vi "Create Sample Clock.vi"(8 "error in (no error)":errorcluster, 11 "DAQmx in":refnum<class "DAQmx.lvclass">) -> (0 "error out":errorcluster, 3 "DAQmx out":refnum<class "DAQmx.lvclass">)   [LabVIEW 2019, in "DAQmx.lvclass"]
uses:
  DAQmx.lvclass
  <resource>/objmgr/daqmx.rc
  <vilib>/DAQmx/configure/timing.llb/DAQmx Timing (Sample Clock).vi
  typedefs/DAQ.Config.Sampling.Sampling--Cluster.ctl
panel:
  out "Sampling":T1={"Fs"=204789.0, "#s"=15753} {"Fs" format="%#_13g"}
  out "Fs (S/s) 3":dbl[](array[numeric]) format="%#_13g"
  out "Fs (S/s) 2":dbl[](array[numeric]) format="%#_13g"
  out "Output.Onboard Buffer":u32[](array[numeric])
  out "Output.Buffer":u32[](array[numeric])
  out "Input.Onboard Buffer":u32[](array[numeric])
  out "Input.Buffer":u32[](array[numeric])
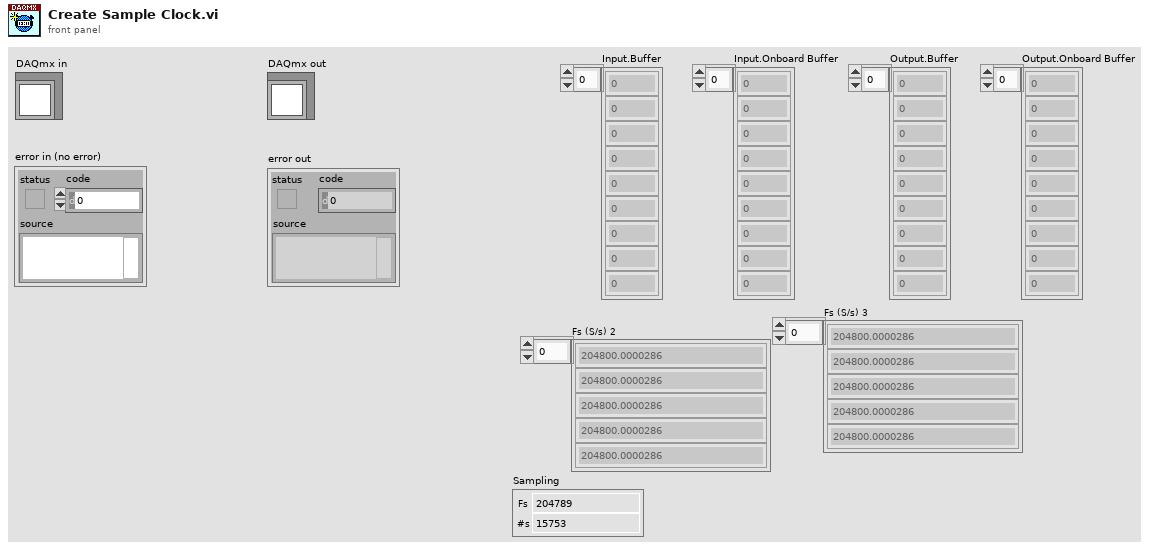
[diagram p1: front panel]
types:
  T1 = typedef "DAQmx.lvclass/DAQ.Config.Sampling.Sampling--Cluster.ctl" = cluster{"Fs":dbl, "#s":i32}
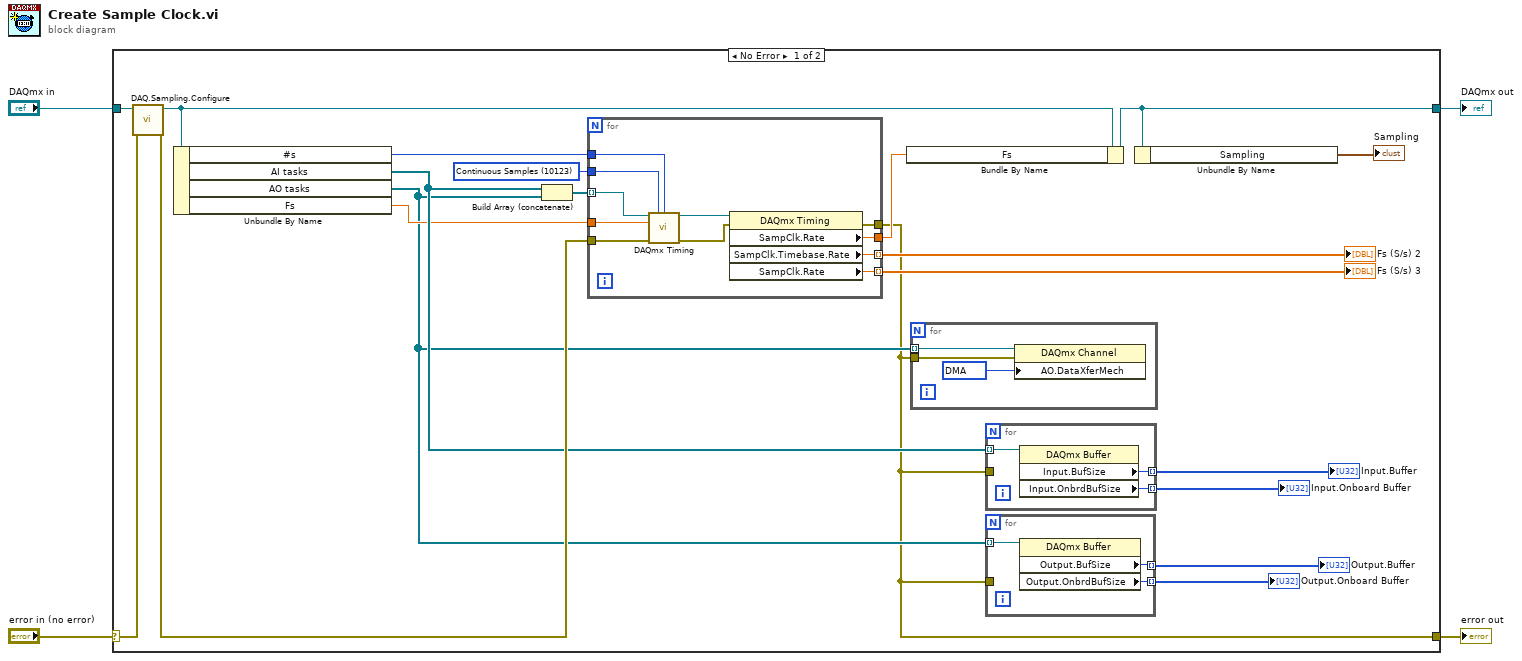
[diagram p0: block diagram]
diagram:
  n1 = case shown="No Error" "error in (no error)" {
    selector: "error in (no error)" -> [w14 w46]
    tunnel: [w5 w46] -> w4
    tunnel: [w9 w45] -> w2
    tunnel: "DAQmx in" -> [w24 w45]
    frame No Error {
      w8 = 10123 items=["Finite Samples"=10178, "Continuous Samples"=10123, "Hardware Timed Single Point"=12522] ("sample mode")
      n2 = call "DAQ.Sampling.Configure.vi"("error in (no error)"=w14, "DAQmx in"=w24) -> ("error out"=w22:errorcluster, "DAQmx out"=w23:refnum<class "DAQmx.lvclass">)  [unwired: 7 in, 1 out]
      n3 = Unbundle By Name(w23) -> ("#s"=w15:i32, "AI tasks"=w16:refnum<k21>[], "AO tasks"=w7:refnum<k21>[], "Fs"=w13:dbl)
      n4 = Build Array (concatenate)(w16, w7) -> (w21:refnum<k21>[])
      n5 = for {
        tunnel: w21 -> [w33] mode=indexing
        tunnel: w13 -> [w32]
        tunnel: w22 -> [w31]
        tunnel: [w35] -> w5
        tunnel: [w37] -> w12
        tunnel: w15 -> [w34]
        tunnel: [w30] -> w11 mode=indexing
        tunnel: [w29] -> w10 mode=indexing
        tunnel: w8 -> [w28]
        n6 = call-poly <vilib>:"DAQmx Timing.vi"("task/channels in"=w33, "sample mode"=w28, "samples per channel"=w34, "rate"=w32, "error in"=w31) -> ("task out"=w38:refnum<k21>, "error out"=w36:errorcluster)  [unwired: 9 in]
        n7 = property class="DAQmx Timing"(reference=w38, error in=w36) -> (error out=w35:errorcluster, "SampClk.Rate"=w37:dbl, "SampClk.Timebase.Rate"=w30:dbl, "SampClk.Rate"=w29:dbl)  [unwired: 1 out]
      }
      "Fs (S/s) 2" <- w11
      "Fs (S/s) 3" <- w10
      n8 = Bundle By Name(cluster=w23, "Fs"=w12) -> (w9:refnum<class "DAQmx.lvclass">)
      n9 = for {
        tunnel: w7 -> [w27] mode=indexing
        tunnel: w5 -> [w26]
        w25 = 10054 items=["DMA"=10054, "Interrupts"=10204, "Programmed I/O"=10264, "USB Bulk"=12590] ("AO.DataXferMech")
        n10 = property class="DAQmx Channel"(reference=w27, error in=w26, "AO.DataXferMech"=w25) -> ()  [unwired: 2 out]
      }
      n11 = for {
        tunnel: w16 -> [w44] mode=indexing
        tunnel: [w43] -> w20 mode=indexing
        tunnel: [w42] -> w19 mode=indexing
        tunnel: w5 -> [_]
        n12 = property class="DAQmx Buffer"(reference=w44) -> ("Input.BufSize"=w43:u32, "Input.OnbrdBufSize"=w42:u32)  [unwired: 1 in, 2 out]
      }
      "Input.Buffer" <- w20
      "Input.Onboard Buffer" <- w19
      n13 = for {
        tunnel: w7 -> [w41] mode=indexing
        tunnel: [w40] -> w18 mode=indexing
        tunnel: [w39] -> w17 mode=indexing
        tunnel: w5 -> [_]
        n14 = property class="DAQmx Buffer"(reference=w41) -> ("Output.BufSize"=w40:u32, "Output.OnbrdBufSize"=w39:u32)  [unwired: 1 in, 2 out]
      }
      "Output.Buffer" <- w18
      "Output.Onboard Buffer" <- w17
      n15 = Unbundle By Name(w9) -> ("Sampling"=→"Sampling":T1)
    }
    frame Error {
    }
  }
  "error out" <- w4
  "DAQmx out" <- w2
